vi "test.vi"() -> ()   [LabVIEW 2020, in "I2C Module.lvlib"]
uses:
  Downloads/I2C Module 1/I2C Module/I2C Module.lvlib
panel:
  out "Waveform Chart":cluster{dbl, dbl}(graph)
  out "SDA":dbl(graph)
  in  "Frequency":dbl
  out "Sine":dbl(graph)
  in  "y":dbl
  out "SCL":dbl(graph)
  in  "Boolean":bool
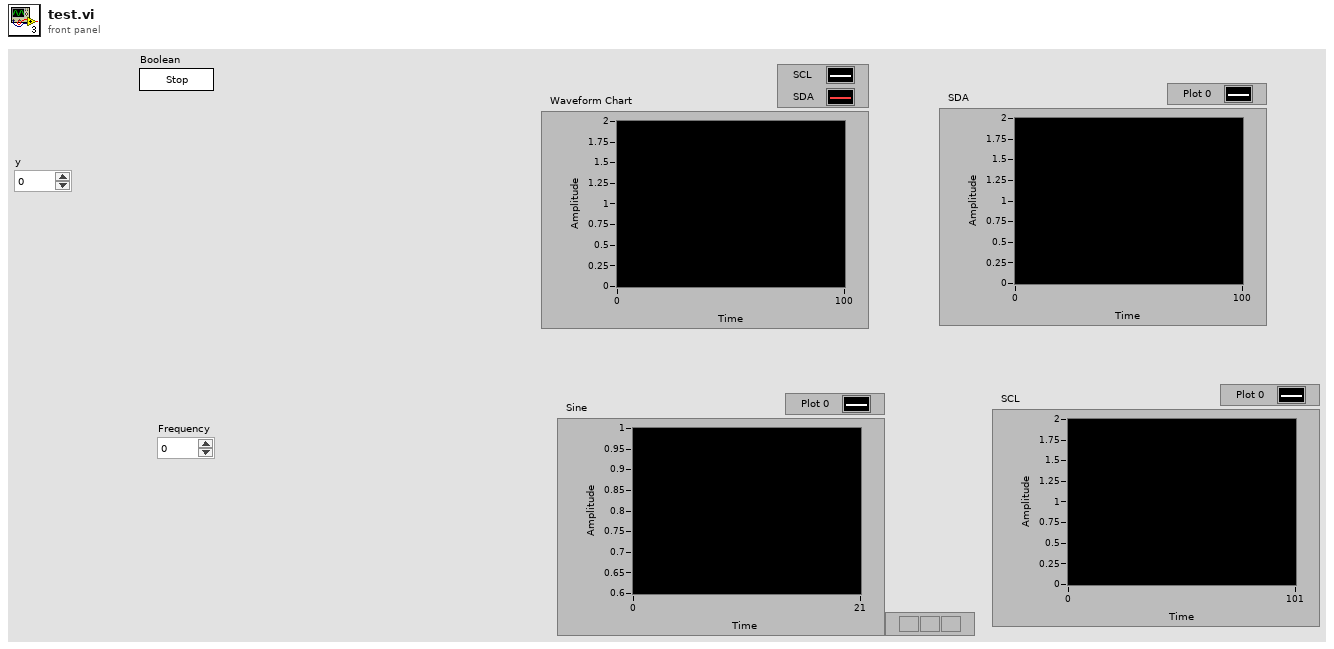
[diagram p1: front panel]
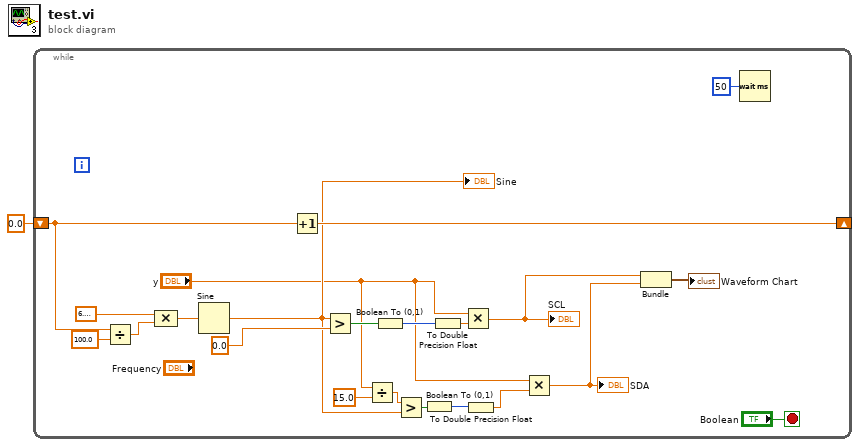
[diagram p0: block diagram]
diagram:
  n1 = while {
    shift-right: [w10] -> _
    shift-left: 0.0 -> [w11]
    stop <- "Boolean" stop-if-true
    n2 = Divide(x=w11, y=100.0) -> (x/y=w21:dbl)
    n3 = Compound Arithmetic op=MULTIPLY(6.283185307179586, w21) -> (w22:dbl)
    n4 = Sine(x=w22) -> (sin(x)=w8:dbl)
    "Sine" <- w8
    n5 = Increment(x=w11) -> (x+1=w10:dbl)
    n6 = Greater?(x=w8, y=0.0) -> (0:w17:bool)
    n7 = Divide(x="y", y=15.0) -> (x/y=w7:dbl)
    n8 = Boolean To (0,1)(Boolean=w17) -> (0, 1=w15:i16)
    n9 = Greater?(x=w7, y=w8) -> (0:w14:bool)
    n10 = Boolean To (0,1)(Boolean=w14) -> (0, 1=w13:i16)
    n11 = To Double Precision Float(number=w15) -> (double precision float=w16:dbl)
    n12 = Multiply(x="y", y=w16) -> (x*y=w4:dbl)
    "SCL" <- w4
    n13 = To Double Precision Float(number=w13) -> (double precision float=w12:dbl)
    n14 = Multiply(x="y", y=w12) -> (x*y=w3:dbl)
    "SDA" <- w3
    n15 = Bundle(w4, w3) -> (→"Waveform Chart":cluster{dbl, dbl})  [unwired: 1 in]
    n16 = Wait (ms)(milliseconds to wait=u32 50) -> ()  [unwired: 1 out]
  }
